vi "Get Matches for all sides.vi"(8 "error in (no error)":errorcluster, 11 "Tile in":refnum<class "Tile.lvclass">) -> (0 "error out":errorcluster, 2 "Matches":u64[](array[numeric]), 3 "Tile out":refnum<class "Tile.lvclass">)   [LabVIEW 2020, in "Tile.lvclass"]
uses:
  Tile.lvclass
  Tile.lvclass/Tile.ctl
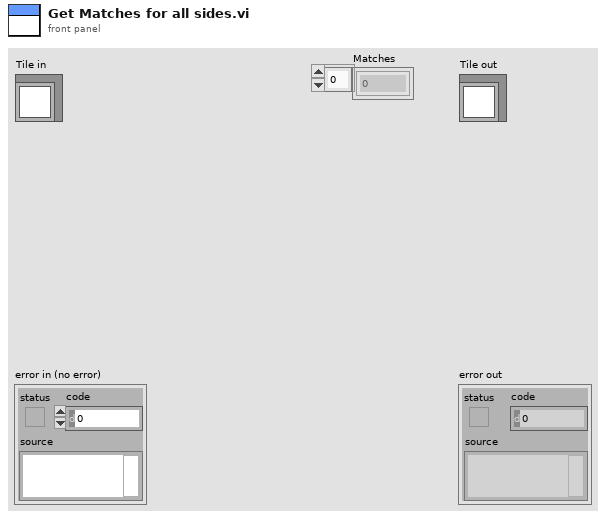
[diagram p1: front panel]
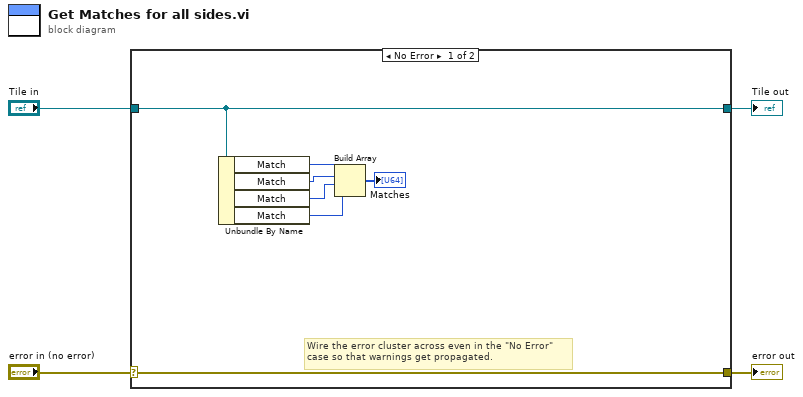
[diagram p0: block diagram]
diagram:
  n1 = case shown="No Error" "error in (no error)" {
    selector: "error in (no error)" -> [w11 w13]
    tunnel: [w11 w13] -> w3
    tunnel: [w10 w12] -> w1
    tunnel: "Tile in" -> [w10 w12]
    frame No Error {
      # "Wire the error cluster across even in the \"No Error\"\ncase so that warnings get propagated."
      n2 = Unbundle By Name(w10) -> ("Match"=w6:u64, "Match"=w7:u64, "Match"=w8:u64, "Match"=w9:u64)
      n3 = Build Array(w6, w7, w8, w9) -> (→"Matches":u64[])
    }
    frame Error {
    }
  }
  "error out" <- w3
  "Tile out" <- w1
